vi "Cleanup.vi"(8 "error in (no error)":errorcluster, 11 "VectoService in":refnum<class "VectoService.lvclass">) -> (0 "error out":errorcluster)   [LabVIEW 2020]
uses:
  VectoService.lvclass
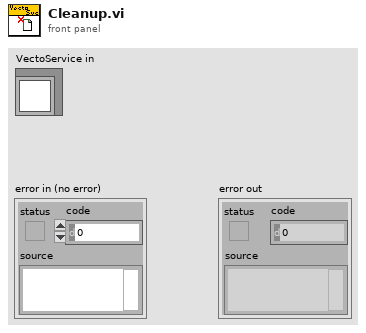
[diagram p1: front panel]
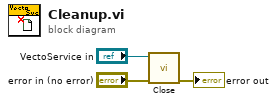
[diagram p0: block diagram]
diagram:
  n1 = call "Close.vi"("error in (no error)"="error in (no error)", "VectoService in"="VectoService in") -> ("error out"=→"error out":errorcluster)  [unwired: 9 in]
